vi "Save Image To Memory.vi"(7 "Save Format":T1, 8 "error in (no error)":errorcluster, 10 "Image":T2) -> (0 "error out":errorcluster, 3 "Encoded Image":u8[](array[numeric]))   [LabVIEW 2020, in "G-Image.lvlib"]
doc: "Saves an image in the selected format and returns the encoded image as a byte array."
uses:
  G-Image.lvlib
  <vilib>/picture/picture.llb/imagedata.ctl
  Controls/Image Save Format.ctl
  <vilib>/Utility/error.llb/Error Cluster From Error Code.vi
  lib/g_image_32.dll
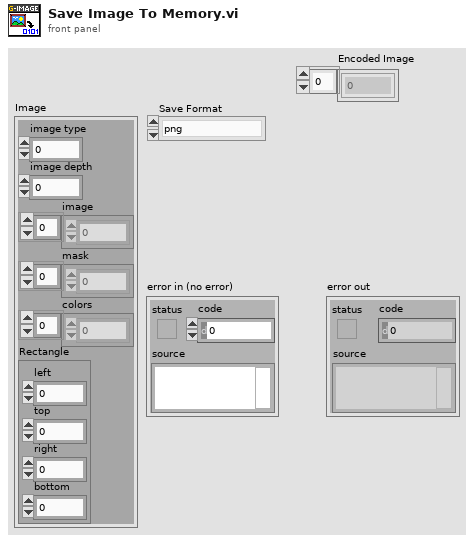
[diagram p1: front panel]
types:
  T1 = typedef "G-Image.lvlib/Image Save Format.ctl" = enum16{"png", "jpg", "bmp", "gif", "tga"}
  T2 = typedef "imagedata.ctl" = cluster{"image type":i32, "image depth":i32, "image":u8[], "mask":u8[], "colors":u32[], "Rectangle":cluster{"left":i16, "top":i16, "right":i16, "bottom":i16}}
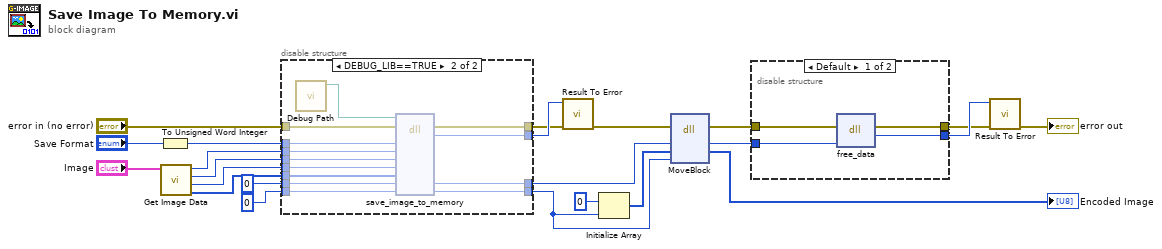
[diagram p0: block diagram]
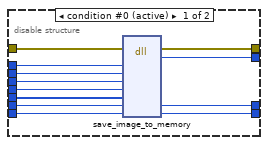
[diagram p2: hidden frame]
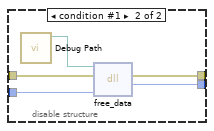
[diagram p3: hidden frame]
diagram:
  n1 = To Unsigned Word Integer(number="Save Format") -> (unsigned 16bit integer=w19:u16)
  n2 = call "Get Image Data.vi"("Image"="Image") -> ("Image (RGBA)"=w1:u8[], "Channels"=w2:i32, "Height"=w3:i32, "Width"=w4:i32)  [unwired: 7 in]
  n3 = disable-structure shown="DEBUG_LIB==TRUE" {
    disable-tunnel: [w35 w48] -> w21
    disable-tunnel: "error in (no error)" -> [w34 w47]
    disable-tunnel: [w33 w46] -> w22
    disable-tunnel: w19 -> [w32 w45]
    disable-tunnel: w4 -> [w31 w44]
    disable-tunnel: w3 -> [w30 w43]
    disable-tunnel: w2 -> [w29 w42]
    disable-tunnel: w1 -> [w28 w41]
    disable-tunnel: [w27 w40] -> w18
    disable-tunnel: [w26 w39] -> w15
    disable-tunnel: i64 0 -> [w25 w38]
    disable-tunnel: 0 -> [w24 w37]
    frame condition #0 (active) {
      n4 = dll-call lib="C:/github/dataflowg/g-image/src/LabVIEW/G-Image/lib/g_image_*.*" fn="save_image_to_memory"(error in=w34, "format"=w32, "width"=w31, "height"=w30, "channels"=w29, "image_data"=w28, "encoded_image"=w25, "encoded_image_count"=w24) -> (error out=w35:errorcluster, "result"=w33:i32, "encoded_image"=w27:i64, "encoded_image_count"=w26:i32)  [unwired: 7 in, 1 out]
    }
    frame condition #1 {
      n5 = call "Debug Path.vi"() -> ("Debug Path"=w36:path)  [unwired: 11 in]
      n6 = dll-call lib="?" fn="save_image_to_memory"(path in=w36, error in=w47, "format"=w45, "width"=w44, "height"=w43, "channels"=w42, "image_data"=w41, "encoded_image"=w38, "encoded_image_count"=w37) -> (error out=w48:errorcluster, "result"=w46:i32, "encoded_image"=w40:i64, "encoded_image_count"=w39:i32)  [unwired: 6 in, 1 out]
    }
  }
  n7 = call "Result To Error.vi"("error in (no error)"=w21, "Result Code"=w22) -> ("error out"=w14:errorcluster)  [unwired: 9 in]
  n8 = Initialize Array(u8 0 ("element"), w15) -> (w16:u8[])
  n9 = dll-call lib="LabVIEW" fn="MoveBlock"(error in=w14, "Address (Pointer)"=w18, "Destination"=w16, "Size"=w15) -> (error out=w9:errorcluster, "Address (Pointer)"=w10:i64, "Destination"=→"Encoded Image":u8[])  [unwired: 4 in, 1 out]
  n10 = disable-structure shown="Default" {
    disable-tunnel: w10 -> [w52 w57]
    disable-tunnel: w9 -> [w51 w56]
    disable-tunnel: [w50 w55] -> w8
    disable-tunnel: [w49 w54] -> w7
    frame condition #0 (active) {
      n11 = dll-call lib="C:/github/dataflowg/g-image/src/LabVIEW/G-Image/lib/g_image_*.*" fn="free_data"(error in=w51, "encoded_image"=w52) -> (error out=w49:errorcluster, "result"=w50:i32)  [unwired: 3 in, 1 out]
    }
    frame condition #1 {
      n12 = call "Debug Path.vi"() -> ("Debug Path"=w53:path)  [unwired: 11 in]
      n13 = dll-call lib="?" fn="free_data"(path in=w53, error in=w56, "encoded_image"=w57) -> (error out=w54:errorcluster, "result"=w55:i32)  [unwired: 2 in, 1 out]
    }
  }
  n14 = call "Result To Error.vi"("error in (no error)"=w7, "Result Code"=w8) -> ("error out"=→"error out":errorcluster)  [unwired: 9 in]
